vi "Resistor set.vi"(7 "Channel  (1: CH1)":u16(ring)=1 items=["CH1"=1, "CH2"=2, "CH3"=3, "CH4"=4], 8 "error in (no error)":errorcluster, 10 "Resistor":dbl, 11 "VISA resource name":refnum<visa-resource-name>) -> (0 "error out":errorcluster, 3 "VISA resource name out":refnum<visa-resource-name>)   [LabVIEW 2020, in "GPP.lvlib"]
uses:
  GPP.lvlib
  Function/VISA_COMMON.ctl
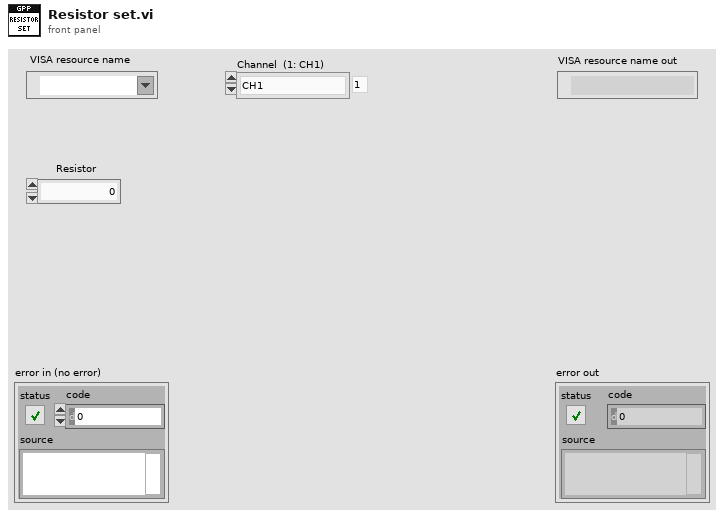
[diagram p1: front panel]
types:
  T1 = typedef "GPP.lvlib/VISA_COMMON.ctl" = enum16{"Initial", "Write CMD", "Read Result", "Read History", "Close"}
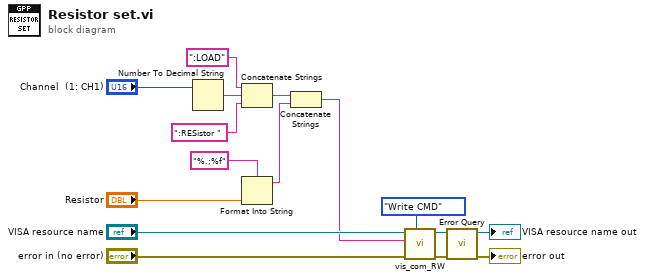
[diagram p0: block diagram]
diagram:
  n1 = Number To Decimal String(number="Channel  (1: CH1)") -> (decimal integer string=w16:string)  [unwired: 1 in]
  n2 = Concatenate Strings(":LOAD", w16, ":RESistor ") -> (w14:string)
  n3 = Format Into String(format string="%.;%f", "Resistor") -> (resulting string=w7:string)  [unwired: 2 in, 1 out]
  n4 = Concatenate Strings(w14, w7) -> (w3:string)
  n5 = call "vis_com_RW.vi"("Funciton"=VISA_COMMON."Write CMD", "error in (no error)"="error in (no error)", "CMD String"=w3, "VISA resource in"="VISA resource name") -> ("error out"=w9:errorcluster, "VISA resource out"=w10:refnum<visa-resource-name>)  [unwired: 5 in, 1 out]
  n6 = call "Error Query.vi"("error in (no error)"=w9, "VISA resource name"=w10) -> ("error out"=→"error out":errorcluster, "VISA resource name out"=→"VISA resource name out":refnum<visa-resource-name>)  [unwired: 6 in, 2 out]
